vi "imagenCam.vi"(4 "Valor Gamma":dbl=1.0 min=1.0 max=2.2, 6 "Ganancia":i64 min=0 max=100, 7 "Exposure":dbl=0.05 min=5e-05 max=0.053229, 8 "tiempo de exposición (ms)":i32, 9 "grupo":string, 10 "nombre":string, 11 "Optional Rectangle":i32[](array[numeric])) -> (1 "Image Pixels (U8)":u8[][](array[numeric]), 2 "Image":T3(plugin-control))   [LabVIEW 2016]
uses:
  <vilib>/vision/driver/IMAQdx.llb/IMAQdx Attribute Type.ctl
  <vilib>/userdefined/High Color/IMAQdx.ctl
  <vilib>/Platform/TimedLoop/XDataNode/timing_clust.ctl
  <vilib>/Platform/TimedLoop/XDataNode/nitl_modes.ctl
  <vilib>/Platform/TimedLoop/XDataNode/wakeup.ctl
  <vilib>/platform/TimedLoop/XDataNode/XDataNode.xnode
  <vilib>/vision/driver/NI_Vision_Acquisition_Software.lvlib
  <vilib>/Platform/TimedLoop/XDataNode/XDNodeRunTimeDep.lvlib
  <resource>/objmgr/imaqdx.rc
  <vilib>/vision/NI_Vision_Development_Module.lvlib
panel:
  out "Attribute Information Array":T2(array[cluster])
  out "Image Pixels (U8) 2":u8[][](array[numeric])
  out "Image 2":T3(plugin-control)
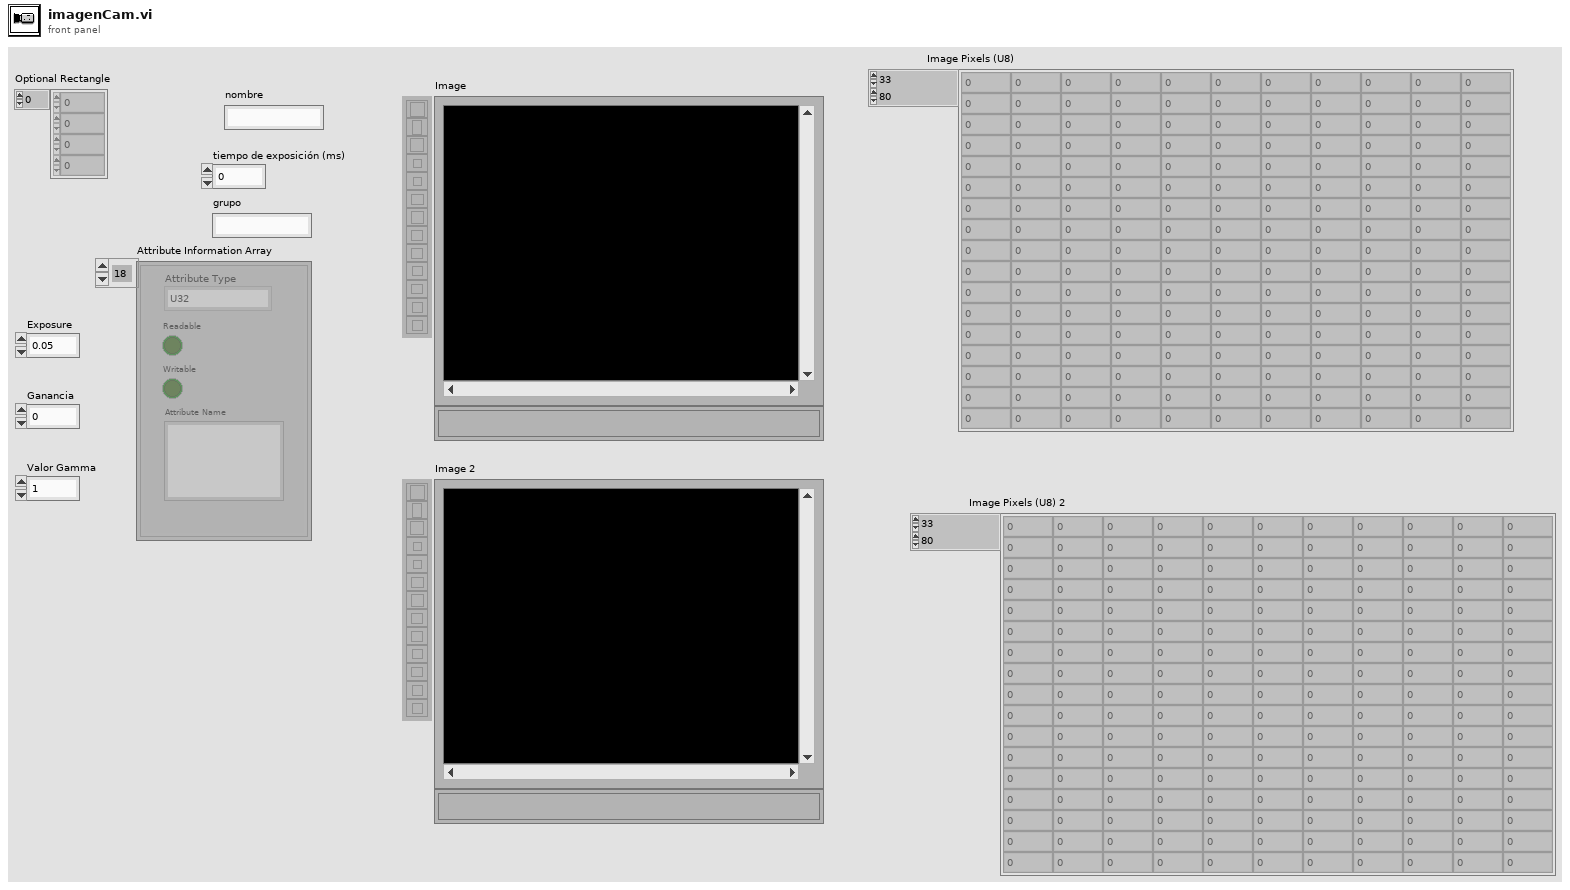
[diagram p1: front panel]
types:
  T1 = typedef "NI_Vision_Acquisition_Software.lvlib/IMAQdx Attribute Type.ctl" = enum32{"U32", "I64", "DBL", "String", "Enum", "Bool", "Command"}
  T2 = cluster{"Attribute Type":T1, "Readable":bool, "Writable":bool, "Attribute Name":string}[]
  T3 = typedef "IMAQ Image.ctl" = refnum<image>
  T4 = enum16{"espejos", "polarizador", "voltaje", "potenciometro y lockin", "CCD"}
  T5 = typedef "IMAQdx.ctl" = refnum<k21>
  T6 = typedef "XDNodeRunTimeDep.lvlib/timing_clust.ctl" = cluster{"Expected End [f-1]":u64, "Actual End [f-1]":u64, "Finished Late? [f-1]":bool, "Expected End [i-1]":u64, "Actual End [i-1]":u64, "Finished Late? [i-1]":bool, "Expected Start [i]":u64, "Actual Start [i]":u64, "Expected Start [f]":u64, "Actual Start [f]":u64, "Source Name":string, "Structure Name":string, "Period":i64, "Deadline":i64, "Offset":i64, "Start":i64, "Priority":i32, "Timeout":i32, "Mode":T7, "Wakeup Reason":T8, "Error":errorcluster, "Source Type":string, "Secondary Source Type":string, "Global End Time":u64, "Global Start Time":u64, "Frame Duration":u64, "Iteration Duration":u64, "Assigned CPU":i32, "I/O Scan Engine Mode":u32}
  T7 = typedef "XDNodeRunTimeDep.lvlib/nitl_modes.ctl" = enum32{"No Change", "Process missed periods, maintain original phase", "Discard missed periods, maintain original phase", "Process missed periods, ignore original phase", "Discard missed periods, ignore original phase"}
  T8 = typedef "XDNodeRunTimeDep.lvlib/wakeup.ctl" = enum32{"Normal", "Aborted", "Asynchronous wakeup", "Timing source error", "Timed loop error", "Timeout"}
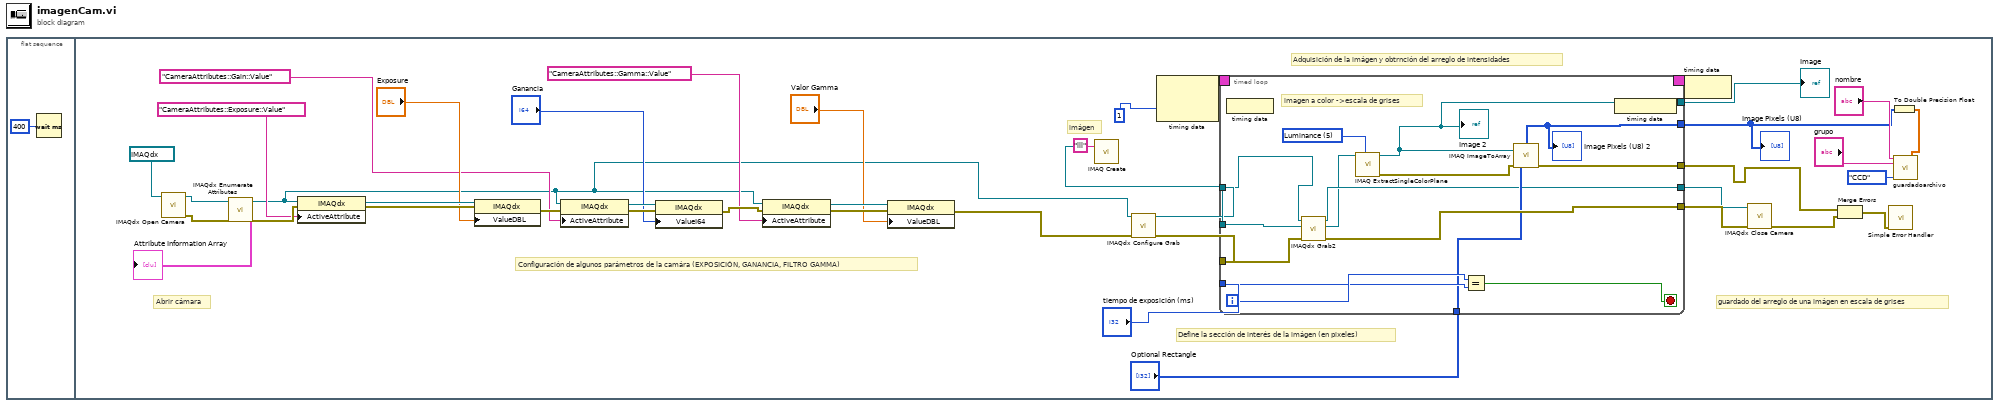
[diagram p0: block diagram]
diagram:
  n1 = flat-sequence {
    frame #0 {
      n2 = Wait (ms)(milliseconds to wait=u32 400) -> ()  [unwired: 1 out]
    }
    frame #1 {
      # "imágen"
      # "Define la sección de interés de la imágen (en pixeles)"
      # "Configuración de algunos parámetros de la camára (EXPOSICIÓN, GANANCIA, FILTRO GAMMA)"
      # "Abrir cámara"
      # "guardado del arreglo de una imágen en escala de grises"
      # "Adquisición de la imágen y obtrnción del arreglo de intensidades"
      n3 = call <vilib>:"IMAQdx Open Camera.vi"("Session In"=T5 "cam4") -> ("error out"=w26:errorcluster, "Session Out"=w7:T5)  [unwired: 9 in]
      n4 = call <vilib>:"IMAQdx Enumerate Attributes.vi"("error in"=w26, "Session In"=w7) -> ("error out"=w24:errorcluster, "Attribute Information Array"=→"Attribute Information Array":T2, "Session Out"=w8:T5)  [unwired: 7 in]
      n5 = property class="IMAQdx"(reference=w8, error in=w24, "ActiveAttribute"="CameraAttributes::Exposure::Value") -> (reference out=w21:T5, error out=w22:errorcluster)
      n6 = property class="IMAQdx"(reference=w21, error in=w22, "ValueDBL"="Exposure") -> (error out=w19:errorcluster)  [unwired: 1 out]
      n7 = property class="IMAQdx"(reference=w8, error in=w19, "ActiveAttribute"="CameraAttributes::Gain::Value") -> (reference out=w17:T5, error out=w16:errorcluster)
      n8 = property class="IMAQdx"(reference=w17, error in=w16, "ValueI64"="Ganancia") -> (error out=w12:errorcluster)  [unwired: 1 out]
      n9 = property class="IMAQdx"(reference=w8, error in=w12, "ActiveAttribute"="CameraAttributes::Gamma::Value") -> (reference out=w14:T5, error out=w13:errorcluster)
      n10 = property class="IMAQdx"(reference=w14, error in=w13, "ValueDBL"="Valor Gamma") -> (error out=w9:errorcluster)  [unwired: 1 out]
      n11 = call "IMAQ Create"("Image Name"="lll") -> ("New Image"=w40:T3)  [unwired: 4 in, 1 out]
      n12 = call <vilib>:"IMAQdx Configure Grab.vi"("error in"=w9, "Session In"=w8) -> ("error out"=w36:errorcluster, "Session Out"=w37:T5)  [unwired: 8 in]
      n13 = node-c288(i64 1 ("Period")) -> (w29:T6)  [unwired: 1 in]
      n14 = timed-loop {
        tunnel: w40 -> [w57]
        tunnel: [w56] -> w39
        tunnel: w37 -> [w47]
        tunnel: [w48] -> w38
        tunnel: w36 -> [w55]
        tunnel: "tiempo de exposición (ms)" -> [w53]
        tunnel: [w49] -> w3
        tunnel: "Optional Rectangle" -> [w51]
        tunnel: [w45] -> w33
        tunnel: [w50] -> w31
        timing: w29 -> [_]
        timing-out: [_] -> w28
        i -> [w54]
        stop <- w52 stop-if-true
        w44 = 5 items=["Red", "Green", "Blue", "Hue", "Saturation", "Luminance", "Value", "Intensity"] ("Color Plane")
        # "imagen a color ->escala de grises"
        n15 = node-c288() -> ()  [unwired: 1 in]
        n16 = call <vilib>:"IMAQdx Grab2.vi"("error in"=w55, "Image In"=w57, "Session In"=w47) -> ("error out"=w56:errorcluster, "Image Out"=w43:T3, "Session Out"=w48:T5)  [unwired: 5 in, 1 out]
        n17 = call "IMAQ ExtractSingleColorPlane"("Color Plane"=w44, "Image Src"=w43) -> ("error out"=w46:errorcluster, "Image Dst Out"=w45:T3)  [unwired: 8 in]
        "Image 2" <- w45
        n18 = Equal?(x=w54, y=w53) -> (x = y?=w52:bool)
        n19 = call "IMAQ ImageToArray"("error in (no error)"=w46, "Optional Rectangle"=w51, "Image"=w45) -> ("error out"=w50:errorcluster, "Image Pixels (U8)"=w49:u8[][])  [unwired: 1 in, 3 out]
        "Image Pixels (U8) 2" <- w49
        n20 = node-c288() -> ()  [unwired: 1 out]
      }
      "Image Pixels (U8)" <- w3
      "Image" <- w33
      n21 = node-c288(w28) -> ()
      n22 = call <vilib>:"IMAQdx Close Camera.vi"("error in"=w39, "Session In"=w38) -> ("error out"=w30:errorcluster)  [unwired: 9 in]
      n23 = Merge Errors(w31, w30) -> (w32:errorcluster)
      n24 = call <vilib>:"Simple Error Handler.vi"("error in (no error)"=w32) -> ()  [unwired: 4 in, 5 out]
      n25 = To Double Precision Float(number=w3) -> (double precision float=w4:dbl[][])
      n26 = call "guardadoarchivo.vi"("nombre"="nombre", "CCD"=w4, "titulo grupo"="grupo", "element"=T4."CCD") -> ()  [unwired: 12 in]
    }
  }
